vi "计算两点之间距离.vi"(10 "Location (Pixel)":cluster{"X":sgl, "Y":sgl}, 11 "Center (Pixels)":cluster{"X":sgl, "Y":sgl}) -> (3 "两点之间距离":sgl)   [LabVIEW 2014]
uses:
  <vilib>/vision/NI_Vision_Development_Module.lvlib
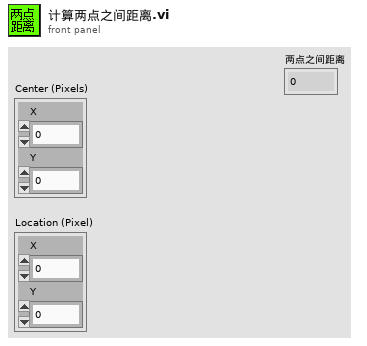
[diagram p1: front panel]
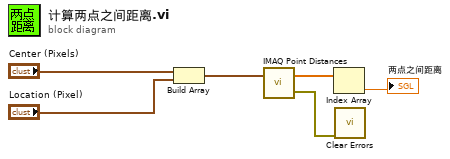
[diagram p0: block diagram]
diagram:
  n1 = Build Array("Center (Pixels)", "Location (Pixel)") -> (w4:cluster{"X":sgl, "Y":sgl}[])
  n2 = call "IMAQ Point Distances"("Points"=w4) -> ("Distances"=w3:sgl[], "error out"=w2:errorcluster)  [unwired: 4 in]
  n3 = Index Array(array=w3) -> (element=→"两点之间距离":sgl)  [unwired: 1 in]
  n4 = call <vilib>:"Clear Errors.vi"("error in (no error)"=w2) -> ()  [unwired: 5 in, 2 out]
